vi "LVCAM Create.vi"(10 "Self Actor":refnum<class "LVCAM.lvclass">, 11 "LVCAM Create in":refnum<class "LVCAM Create.lvclass">) -> (0 "error out":errorcluster, 3 "LVCAM Create out":refnum<class "LVCAM Create.lvclass">)   [LabVIEW 2021, in "LVCAM.lvlib" / "LVCAM Create.lvclass"]
uses:
  LVCAM Create.lvclass
  LVCAM/LVCAM.lvclass
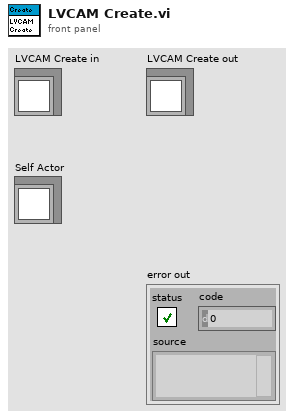
[diagram p1: front panel]
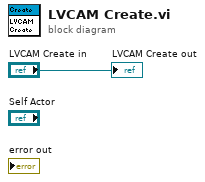
[diagram p0: block diagram]
diagram:
  "LVCAM Create out" <- "LVCAM Create in"
